vi "WSVCAP SHL Host TL RFFE Write - Multiple DUTs - Common Data.vi"(0 "Data Out":string, 11 "error in":errorcluster, 13 "DUT Mask (All)":bool[](array[boolean])=[TRUE, TRUE, TRUE, TRUE, TRUE, TRUE, TRUE, TRUE, TRUE, TRUE, TRUE, TRUE, TRUE, TRUE, TRUE, TRUE, TRUE, TRUE, TRUE, TRUE, TRUE, TRUE, TRUE, TRUE, TRUE, TRUE, TRUE, TRUE, TRUE, TRUE, TRUE, TRUE, TRUE, TRUE, TRUE, TRUE], 14 "Log (T)":bool=TRUE) -> (15 "error out":errorcluster)   [LabVIEW 2012]
panel:
  out "Socket Mask":u64=1 format="%02x"
  out "RFFE Data Out [U8]":u8[][](array[numeric]) format="%02x"
  # "DUT 01"
  # "DUT 02"
  # "DUT 03"
  # "DUT 04"
  # "DUT 05"
  # "DUT 06"
  # "DUT 07"
  # "DUT 08"
  # "DUT 09"
  # "DUT 10"
  # "DUT 11"
  # "DUT 12"
  # "DUT 13"
  # "DUT 14"
  # "DUT 15"
  # "DUT 16"
  # "DUT 17"
  # "DUT 18"
  # "DUT 19"
  # "DUT 20"
  # "DUT 21"
  # "DUT 22"
  # "DUT 23"
  # "DUT 24"
  # "DUT 25"
  # "DUT 26"
  # "DUT 27"
  # "DUT 28"
  # "DUT 29"
  # "DUT 30"
  # "DUT 31"
  # "DUT 32"
  # "DUT 33"
  # "DUT 34"
  # "DUT 35"
  # "DUT 36"
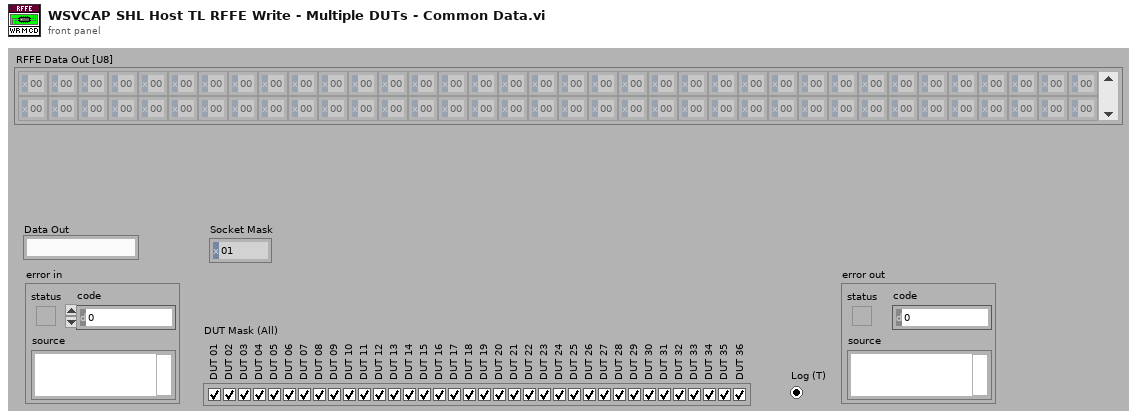
[diagram p1: front panel]
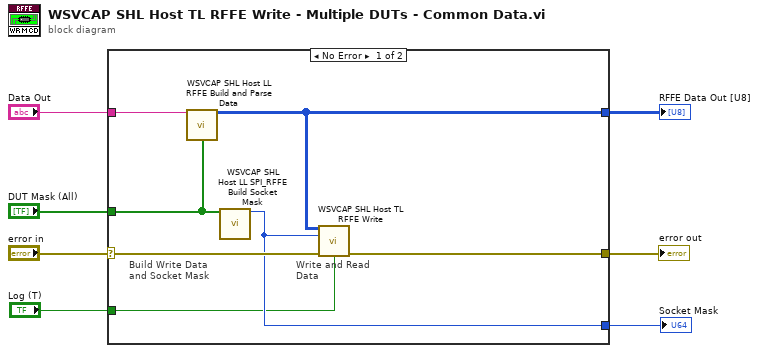
[diagram p0: block diagram]
diagram:
  n1 = case shown="No Error" "error in" {
    selector: "error in" -> [w13 _]
    tunnel: [w14 _] -> w7
    tunnel: "Data Out" -> [w12 _]
    tunnel: [w10 _] -> w4
    tunnel: [w9 _] -> w3
    tunnel: "DUT Mask (All)" -> [w11 _]
    tunnel: "Log (T)" -> [w8 _]
    frame No Error {
      # "Write and Read\nData"
      # "Build Write Data and Socket Mask"
      n2 = call "WSVCAP SHL Host LL RFFE Build and Parse Data.vi"("Data Out"=w12, "DUT Mask (All)"=w11) -> ("RFFE Data Out [U8]"=w10:u8[][])  [unwired: 10 in, 3 out]
      n3 = call "WSVCAP SHL Host LL SPI_RFFE Build Socket Mask.vi"("DUT Mask"=w11) -> ("Socket Mask [U64]"=w9:u64)  [unwired: 14 in]
      n4 = call "WSVCAP SHL Host TL RFFE Write.vi"("RFFE Data Out"=w10, "Socket Mask"=w9, "error in"=w13, "Log (T)"=w8) -> ("error out"=w14:errorcluster)  [unwired: 11 in]
    }
    frame Error {
    }
  }
  "error out" <- w7
  "RFFE Data Out [U8]" <- w4
  "Socket Mask" <- w3
